vi "AngleFilmVariable.vi"() -> ()   [LabVIEW 2015]
panel:
  out "Angle":dbl
  out "Film Height":dbl
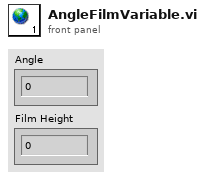
[diagram p1: front panel]
diagram:
